vi "Save Project.vi"(8 "error in (no error)":errorcluster, 11 "Project Sync Tools in":refnum<class "Project Sync Tools.lvclass">) -> (0 "error out":errorcluster, 3 "Project Sync Tools out":refnum<class "Project Sync Tools.lvclass">)   [LabVIEW 2019, in "Project Sync Tools.lvclass"]
uses:
  Project Sync Tools.lvclass
  Project Sync Tools.lvclass/Project Sync Tools.ctl
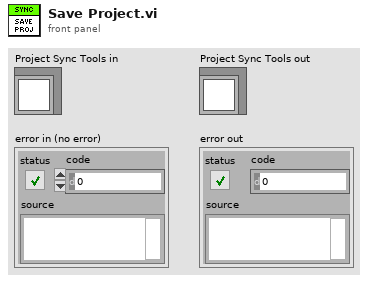
[diagram p1: front panel]
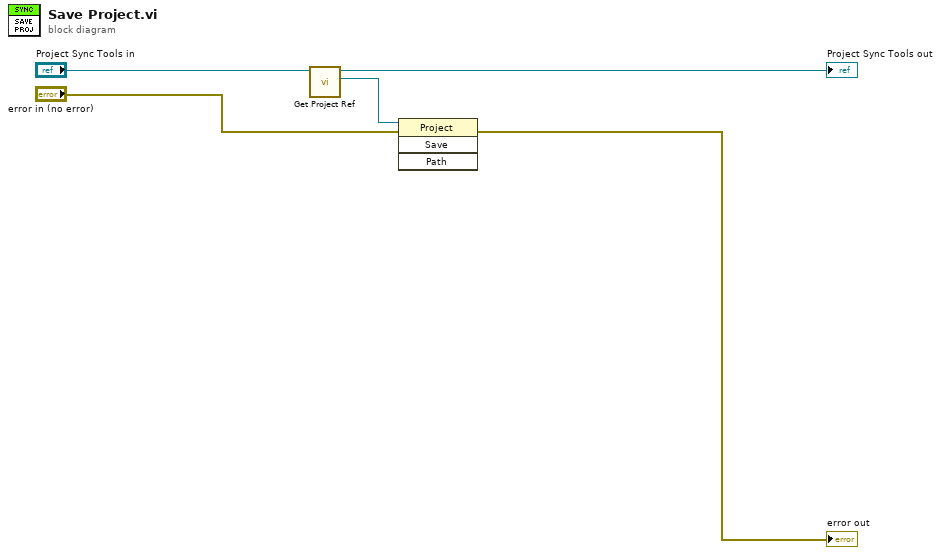
[diagram p0: block diagram]
diagram:
  n1 = call "Get Project Ref.vi"("CD Build Tools in"="Project Sync Tools in") -> ("Project Ref"=w2:refnum<vi>, "CD Build Tools out"=→"Project Sync Tools out":refnum<class "Project Sync Tools.lvclass">)  [unwired: 9 in]
  n2 = invoke class="Project" method="Save"(reference=w2, error in="error in (no error)") -> (error out=→"error out":errorcluster)  [unwired: 2 in, 3 out]
